vi "sub2.vi"() -> (2 "String":string)   [LabVIEW 2013]
panel:
  in  "idle":bool
  in  "stop":bool
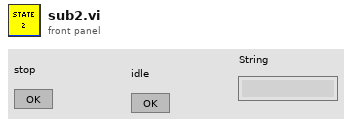
[diagram p1: front panel]
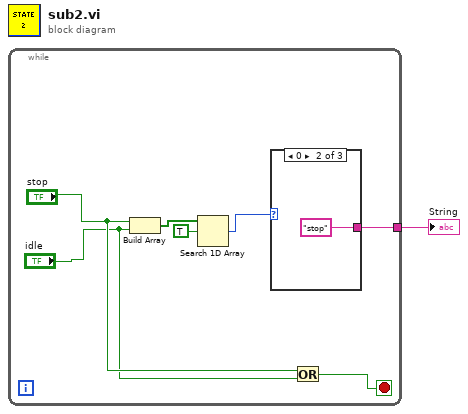
[diagram p0: block diagram]
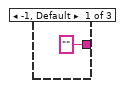
[diagram p2: hidden frame]
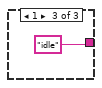
[diagram p3: hidden frame]
diagram:
  n1 = while {
    tunnel: [w4] -> w1
    stop <- w8 stop-if-true
    n2 = Build Array("stop", "idle") -> (w7:bool[])
    n3 = Search 1D Array(1D array=w7, element=TRUE) -> (index of element=w5:i32)  [unwired: 1 in]
    n4 = case shown="0" w5 {
      tunnel: ["" "stop" "idle"] -> w4
      frame -1, Default {
      }
      frame 0 {
      }
      frame 1 {
      }
    }
    n5 = Or(x="stop", y="idle") -> (x .or. y?=w8:bool)
  }
  "String" <- w1
